vi "CRYGet Graph Data in Graph Sub.vi"(6 "Index":i32[](array[numeric]), 7 "sOption":string, 8 "Data Names":string[](array[string]), 9 "sGraphType":string, 10 "Legend Refnum":refnum<vi>, 11 "Type In":enum16{"Curves", "Values", "Results", "WFM"}(ring)) -> (0 "Names Out":string[](array[string]), 1 "bResult":bool, 2 "Rows":i32[](array[numeric]), 3 "Type Out":enum16{"Curves", "Values", "Results", "WFM"}(ring), 5 "bSameRemainReplot":bool)   [LabVIEW 2013]
uses:
  CRYStepSetup/CRYStepSetup Global.vi
  CRYCurveLibrary/Global/CRYCurve Library Global.vi
  CRYMainGlobal.vi
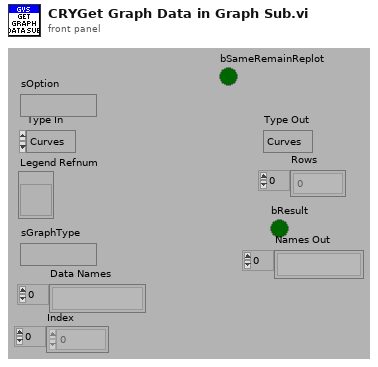
[diagram p1: front panel]
types:
  T1 = cluster{"CurveOld":string[], "ValueOld":string[], "ResultOld":string[], "WFMOld":string[], "CurveNew":string[], "ValueNew":string[], "ResultNew":string[], "WFMNew":string[]}
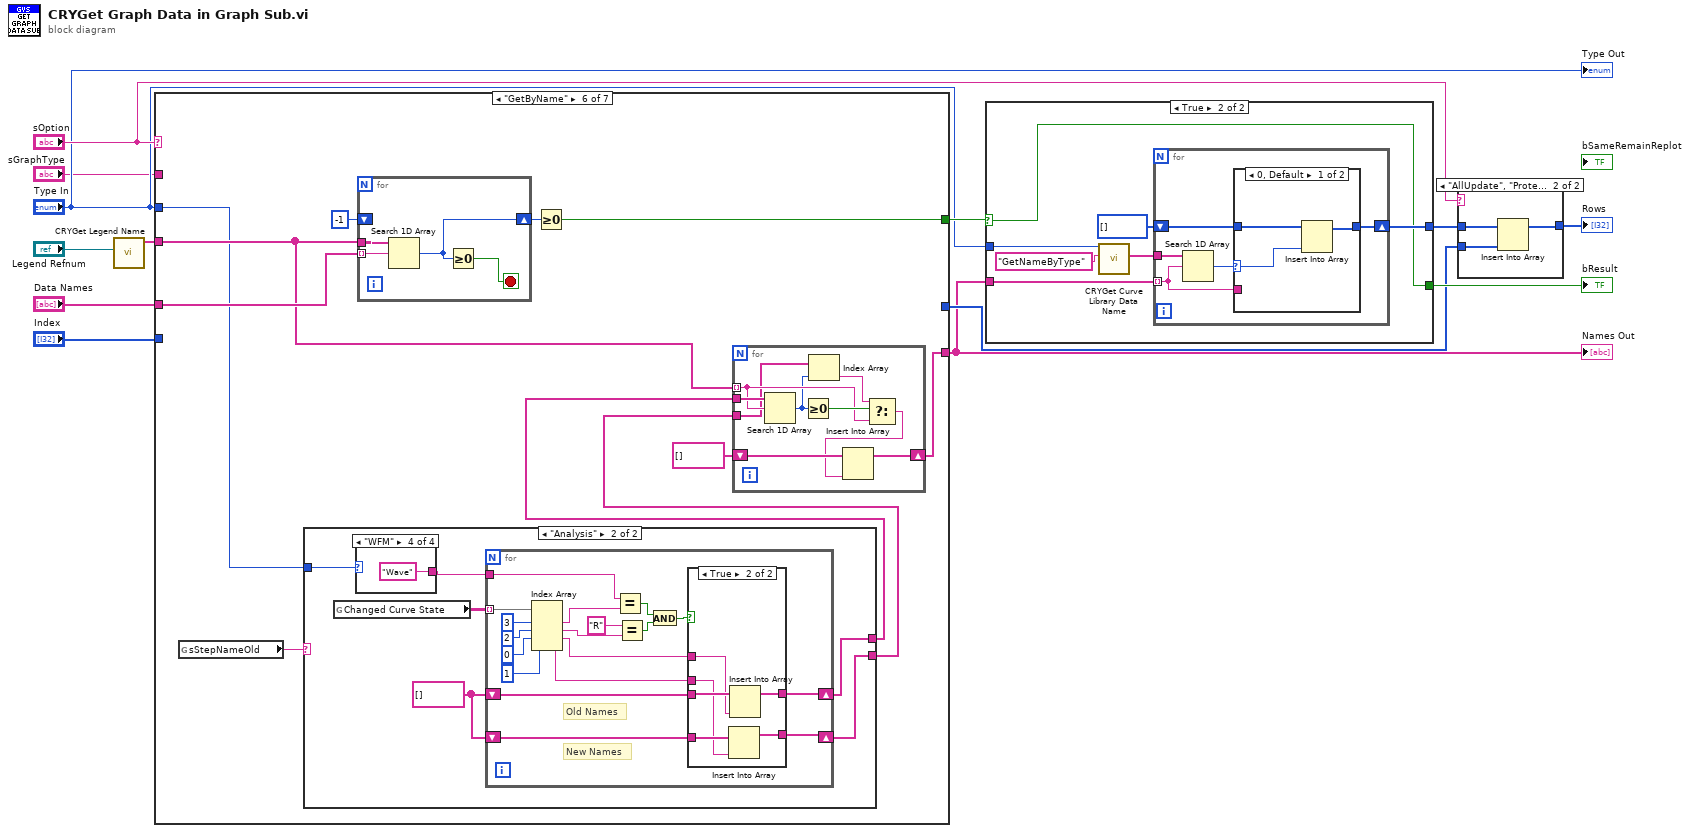
[diagram p0: block diagram]
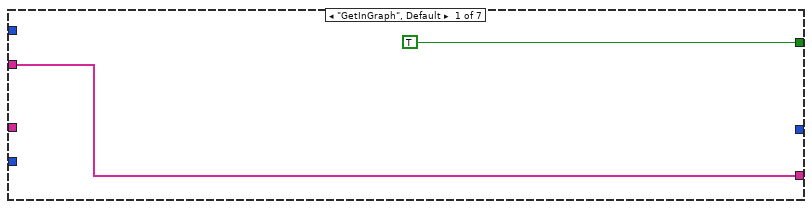
[diagram p3: hidden frame]
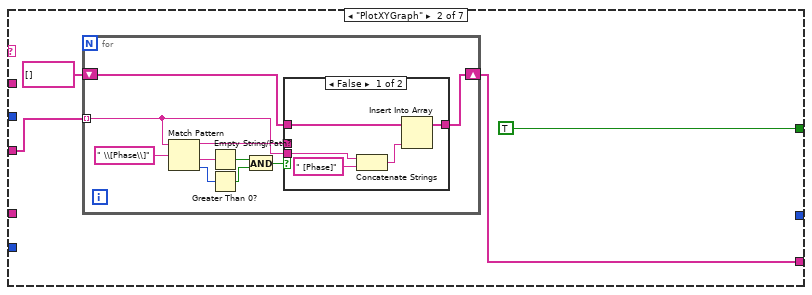
[diagram p4: hidden frame]
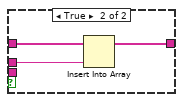
[diagram p5: hidden frame]
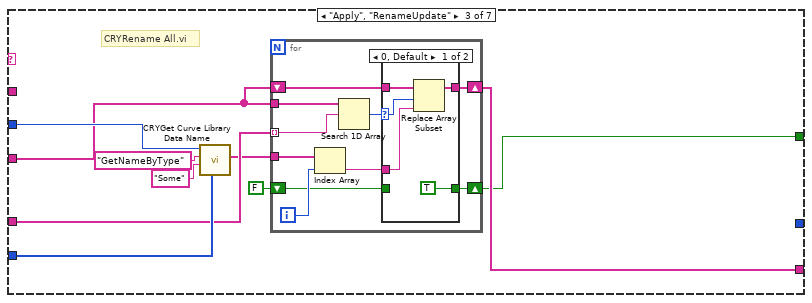
[diagram p6: hidden frame]
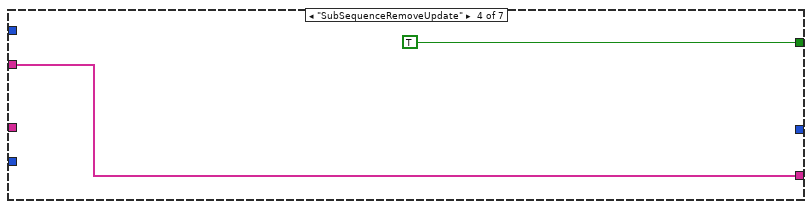
[diagram p8: hidden frame]
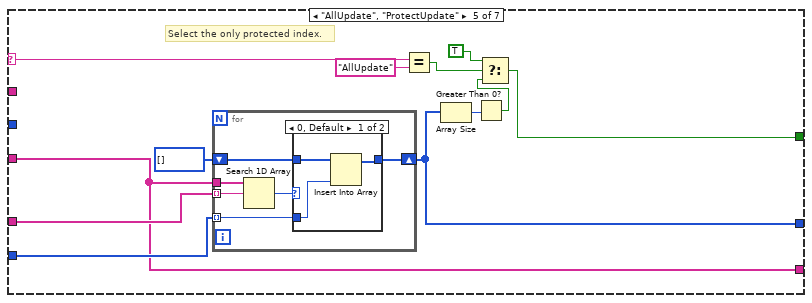
[diagram p9: hidden frame]
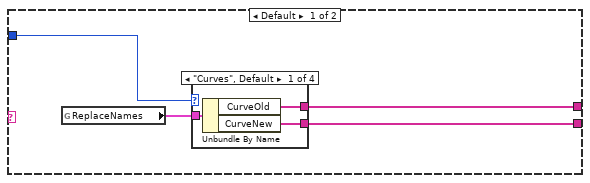
[diagram p11: hidden frame]
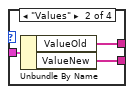
[diagram p12: hidden frame]
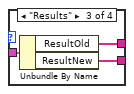
[diagram p13: hidden frame]
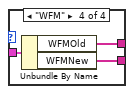
[diagram p14: hidden frame]
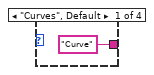
[diagram p15: hidden frame]
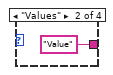
[diagram p16: hidden frame]
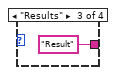
[diagram p17: hidden frame]
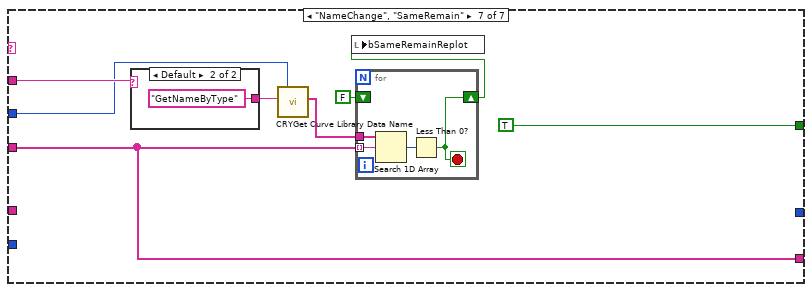
[diagram p19: hidden frame]
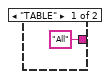
[diagram p20: hidden frame]
diagram:
  n1 = call "CRYGet Legend Name.vi"("MCListbox Refnum"="Legend Refnum") -> ("Names Out"=w9:string[])  [unwired: 2 in, 8 out]
  n2 = case shown="\"GetByName\"" "sOption" {
    selector: "sOption" -> [_ _ _ _ w70 _ _]
    tunnel: "Data Names" -> [_ _ w42 _ w78 w98 _]
    tunnel: w9 -> [w14 w17 w41 w65 w68 w95 w165]
    tunnel: [TRUE TRUE w38 TRUE w73 w96 TRUE] -> w10
    tunnel: "Type In" -> [_ _ w45 _ _ w91 w166]
    tunnel: "Index" -> [_ _ w44 _ w77 _ _]
    tunnel: [_ _ _ _ w67 _ _] -> w4
    tunnel: "sGraphType" -> [_ _ _ _ _ _ w167]
    tunnel: [w14 w16 w43 w65 w68 w93 w165] -> w2
    frame "GetInGraph", Default {
    }
    frame "PlotXYGraph" {
      n3 = for {
        shift-right: [w21] -> w16
        shift-left: string[] [] -> [w22]
        tunnel: w17 -> [w20] mode=indexing
        n4 = Match Pattern(string=w20, regular expression=" \\[Phase\\]") -> (before substring=w23:string, after substring=w26:string, offset past match=w27:i32)  [unwired: 1 in, 1 out]
        n5 = Empty String/Path?(string/path=w26) -> (empty?=w28:bool)
        n6 = Greater Than 0?(x=w27) -> (x > 0?=w29:bool)
        n7 = And(x=w28, y=w29) -> (x .and. y?=w24:bool)
        n8 = case shown="False" w24 {
          tunnel: w23 -> [_ w35]
          tunnel: w22 -> [w34 w37]
          tunnel: w20 -> [w31 _]
          tunnel: [w32 w36] -> w21
          frame False {
            n9 = Concatenate Strings(w31, " [Phase]" ("regular expression")) -> (w30:string)
            n10 = Insert Into Array(array=w34, new element=w30) -> (w32:string[])  [unwired: 1 in]
          }
          frame True {
            n11 = Insert Into Array(array=w37, new element=w35) -> (w36:string[])  [unwired: 1 in]
          }
        }
      }
    }
    frame "Apply", "RenameUpdate" {
      # "CRYRename All.vi"
      n12 = call "CRYGet Curve Library Data Name.vi"("nData"=w44, "sOption"="Some", "sAction"="GetNameByType", "Type"=w45) -> ("sNames"=w40:string[])  [unwired: 2 in, 5 out]
      n13 = for {
        tunnel: w42 -> [w53] mode=indexing
        tunnel: w41 -> [w57]
        shift-right: [w54] -> w43
        shift-left: w41 -> [w55]
        tunnel: w40 -> [w52]
        shift-right: [w48] -> w38
        shift-left: FALSE -> [w49]
        i -> [w51]
        n14 = Index Array(array=w52, index=w51) -> (element=w50:string)
        n15 = Search 1D Array(1D array=w57, element=w53) -> (index of element=w56:i32)  [unwired: 1 in]
        n16 = case shown="0, Default" w56 {
          selector: w56 -> [w59 _]
          tunnel: w55 -> [w62 w64]
          tunnel: [w61 w64] -> w54
          tunnel: w50 -> [w60 _]
          tunnel: w49 -> [_ w63]
          tunnel: [TRUE w63] -> w48
          frame 0, Default {
            n17 = Replace Array Subset(array=w62, new element=w60, index=w59) -> (w61:string[])
          }
          frame -1 {
          }
        }
      }
    }
    frame "SubSequenceRemoveUpdate" {
    }
    frame "AllUpdate", "ProtectUpdate" {
      # "Select the only protected index."
      n18 = for {
        tunnel: w78 -> [w83] mode=indexing
        tunnel: w68 -> [w84]
        shift-right: [w81] -> w67
        shift-left: i32[] [] -> [w82]
        tunnel: w77 -> [w79] mode=indexing
        n19 = Search 1D Array(1D array=w84, element=w83) -> (index of element=w80:i32)  [unwired: 1 out]
        n20 = case shown="0, Default" w80 {
          tunnel: [w86 w88] -> w81
          tunnel: w82 -> [w87 w88]
          tunnel: w79 -> [w85 _]
          frame 0, Default {
            n21 = Insert Into Array(array=w87, new element=w85) -> (w86:i32[])  [unwired: 1 in]
          }
          frame -1 {
          }
        }
      }
      n22 = Equal?(x=w70, y="AllUpdate") -> (x = y?=w69:bool)
      n23 = Array Size(array=w67) -> (size(s)=w72:i32)
      n24 = Greater Than 0?(x=w72) -> (x > 0?=w71:bool)
      n25 = Select(t=TRUE, s=w69, f=w71) -> (s? t:f=w73:bool)
    }
    frame "GetByName" {
      n26 = global read "CRYStepSetup Global.vi" "sStepNameOld"() -> (w92:string)
      n27 = case shown="\"Analysis\"" w92 {
        tunnel: w91 -> [w102 w119]
        tunnel: [w101 w117] -> w90
        tunnel: [w100 w116] -> w89
        frame Default {
          n28 = global read "CRYCurve Library Global.vi" "ReplaceNames"() -> (w103:T1)
          n29 = case shown="\"Curves\", Default" w102 {
            tunnel: w103 -> [w106 w109 w112 w115]
            tunnel: [w105 w108 w111 w114] -> w101
            tunnel: [w104 w107 w110 w113] -> w100
            frame "Curves", Default {
              n30 = Unbundle By Name(w106) -> ("CurveOld"=w105:string[], "CurveNew"=w104:string[])
            }
            frame "Values" {
              n31 = Unbundle By Name(w109) -> ("ValueOld"=w108:string[], "ValueNew"=w107:string[])
            }
            frame "Results" {
              n32 = Unbundle By Name(w112) -> ("ResultOld"=w111:string[], "ResultNew"=w110:string[])
            }
            frame "WFM" {
              n33 = Unbundle By Name(w115) -> ("WFMOld"=w114:string[], "WFMNew"=w113:string[])
            }
          }
        }
        frame "Analysis" {
          w120 = string[] [] ("Changed Curve State")
          n34 = global read "CRYMainGlobal.vi" "Changed Curve State"() -> (w121:string[][])
          n35 = case shown="\"WFM\"" w119 {
            tunnel: ["Curve" ("Custom Curve Names") "Value" ("Custom Curve Names") "Result" ("Custom Curve Names") "Wave" ("Custom Curve Names")] -> w118
            frame "Curves", Default {
            }
            frame "Values" {
            }
            frame "Results" {
            }
            frame "WFM" {
            }
          }
          n36 = for {
            tunnel: w121 -> [w139] mode=indexing
            shift-right: [w129] -> w117
            shift-left: w120 -> [w130]
            shift-right: [w127] -> w116
            shift-left: w120 -> [w128]
            tunnel: w118 -> [w126]
            # "New Names"
            # "Old Names"
            n37 = Index Array(array=w139, index #1=3 ("index"), index #2=2 ("index"), index #3=0 ("index"), index #4=1 ("index")) -> (element #1=w138:string, element #2=w137:string, element #3=w132:string, element #4=w131:string)
            n38 = Equal?(x=w126, y=w138) -> (x = y?=w135:bool)
            n39 = Equal?(x="R", y=w137) -> (x = y?=w134:bool)
            n40 = And(x=w135, y=w134) -> (x .and. y?=w133:bool)
            n41 = case shown="True" w133 {
              tunnel: w132 -> [_ w147]
              tunnel: w131 -> [_ w146]
              tunnel: w130 -> [w145 w151]
              tunnel: [w145 w150] -> w129
              tunnel: w128 -> [w144 w149]
              tunnel: [w144 w148] -> w127
              frame False {
              }
              frame True {
                n42 = Insert Into Array(array=w149, new element=w146) -> (w148:string[])  [unwired: 1 in]
                n43 = Insert Into Array(array=w151, new element=w147) -> (w150:string[])  [unwired: 1 in]
              }
            }
          }
        }
      }
      n44 = for {
        tunnel: w98 -> [w163] mode=indexing
        tunnel: w95 -> [w164]
        shift-right: [w161] -> w97
        shift-left: -1 ("index of element") -> [_]
        stop <- w162 stop-if-true
        n45 = Search 1D Array(1D array=w164, element=w163) -> (index of element=w161:i32)  [unwired: 1 out]
        n46 = Greater Or Equal To 0?(x=w161) -> (x >= 0?=w162:bool)
      }
      n47 = Greater Or Equal To 0?(x=w97) -> (x >= 0?=w96:bool)
      n48 = for {
        tunnel: w95 -> [w158] mode=indexing
        tunnel: w90 -> [w160]
        tunnel: w89 -> [w153]
        shift-right: [w155] -> w93
        shift-left: string[] [] ("WFMNew") -> [w157]
        n49 = Search 1D Array(1D array=w160, element=w158) -> (index of element=w154:i32)  [unwired: 1 out]
        n50 = Greater Or Equal To 0?(x=w154) -> (x >= 0?=w159:bool)
        n51 = Index Array(array=w153, index=w154) -> (element=w152:string)
        n52 = Select(t=w152, s=w159, f=w158) -> (s? t:f=w156:string)
        n53 = Insert Into Array(array=w157, new element=w156) -> (w155:string[])  [unwired: 1 in]
      }
    }
    frame "NameChange", "SameRemain" {
      n54 = case shown="Default" w167 {
        tunnel: ["All" ("sAction") "GetNameByType" ("sAction")] -> w172
        frame "TABLE" {
        }
        frame Default {
        }
      }
      n55 = call "CRYGet Curve Library Data Name.vi"("sAction"=w172, "Type"=w166) -> ("sNames"=w168:string[])  [unwired: 4 in, 5 out]
      n56 = for {
        tunnel: w168 -> [w176]
        tunnel: w165 -> [w175] mode=indexing
        shift-right: [w177] -> w169
        shift-left: FALSE -> [_]
        stop <- w177 stop-if-true
        n57 = Search 1D Array(1D array=w176, element=w175) -> (index of element=w178:i32)  [unwired: 1 out]
        n58 = Less Than 0?(x=w178) -> (x < 0?=w177:bool)
      }
      n59 = local write "bSameRemainReplot"(w169) -> ()
    }
  }
  "Names Out" <- w2
  n60 = case shown="True" w10 {
    selector: w10 -> [w179 w181]
    tunnel: w2 -> [_ w186]
    tunnel: "Type In" -> [_ w184]
    tunnel: [i32[] [] w182] -> w7
    tunnel: [w179 w181] -> w12
    frame False {
    }
    frame True {
      n61 = call "CRYGet Curve Library Data Name.vi"("sAction"="GetNameByType", "Type"=w184) -> ("sNames"=w185:string[])  [unwired: 4 in, 5 out]
      n62 = for {
        tunnel: w186 -> [w188] mode=indexing
        tunnel: w185 -> [w192]
        shift-right: [w189] -> w182
        shift-left: i32[] [] -> [w190]
        n63 = Search 1D Array(1D array=w192, element=w188) -> (index of element=w191:i32)  [unwired: 1 in]
        n64 = case shown="0, Default" w191 {
          selector: w191 -> [w195 _]
          tunnel: [w193 w196] -> w189
          tunnel: w190 -> [w194 w196]
          tunnel: w188 -> [_ _]
          frame 0, Default {
            n65 = Insert Into Array(array=w194, new element=w195) -> (w193:i32[])  [unwired: 1 in]
          }
          frame -1 {
          }
        }
      }
    }
  }
  "bResult" <- w12
  n66 = case shown="\"AllUpdate\", \"ProtectUpdate\"" "sOption" {
    tunnel: [w197 w198] -> w1
    tunnel: w7 -> [w197 w200]
    tunnel: w4 -> [_ w199]
    frame Default {
    }
    frame "AllUpdate", "ProtectUpdate" {
      n67 = Insert Into Array(array=w200, new element=w199) -> (w198:i32[])  [unwired: 1 in]
    }
  }
  "Rows" <- w1
  "Type Out" <- "Type In"
